vi "Login.vi"(0 "reference in":refnum<class "Login_Dialog.lvclass">, 11 "error in (no error)":errorcluster) -> (4 "reference in":refnum<class "Login_Dialog.lvclass">, 6 "User":string, 8 "Valid":bool, 10 "Rights":string[](array[string]), 13 "Password":string, 14 "Cancelled":bool, 15 "error out":errorcluster)   [LabVIEW 2022 SP3, in "Login_Dialog.lvlib" / "Login_Dialog.lvclass"]
uses:
  Login_Dialog.lvclass
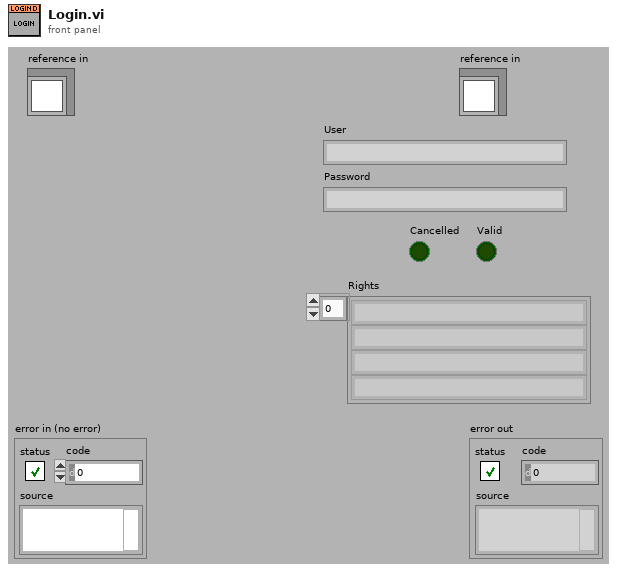
[diagram p1: front panel]
types:
  T1 = typedef "Login_Dialog.lvlib/Login_Dialog.lvclass/ObjectAttributes.ctl" = cluster{"Config":T2, "User":string, "LoggedIn":bool, "Users":string[][]}
  T2 = typedef "Login_Dialog.lvlib/Login_Dialog.lvclass/Config.ctl" = cluster{"default":string}
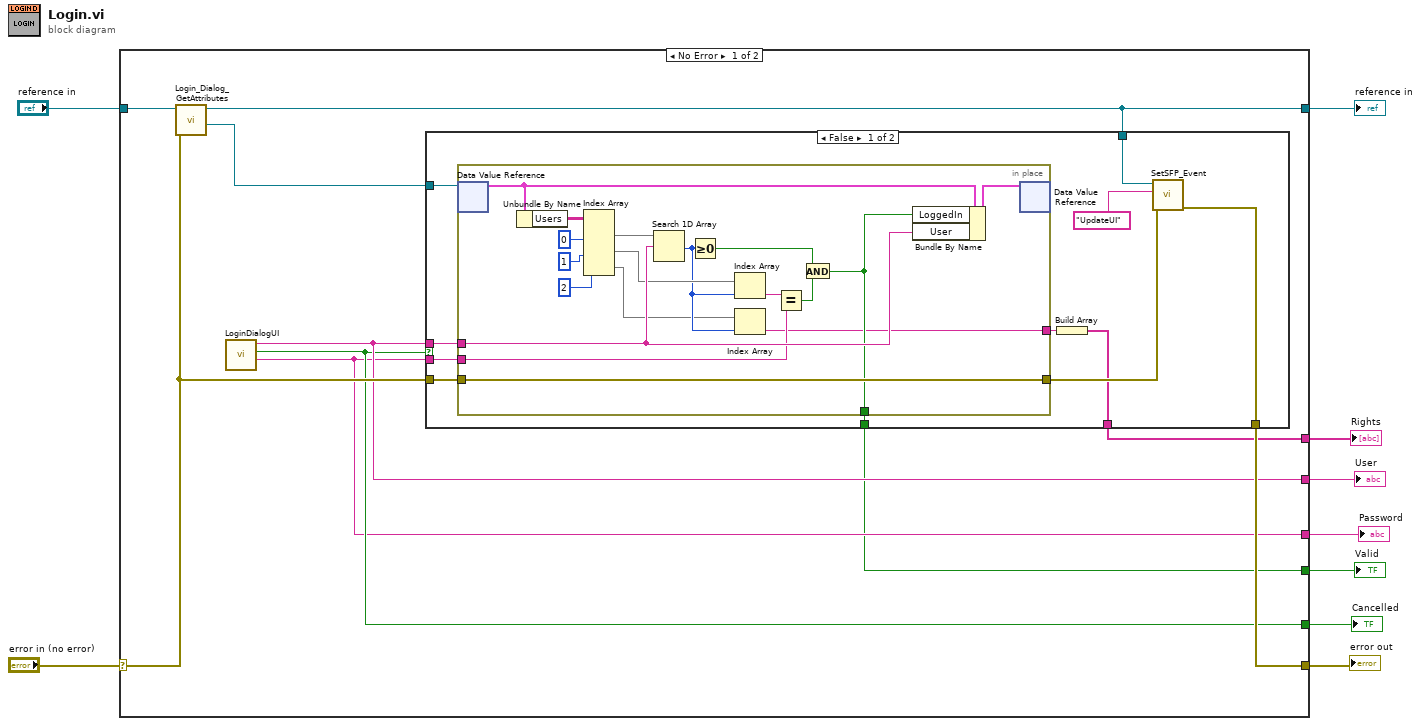
[diagram p0: block diagram]
diagram:
  n1 = case shown="No Error" "error in (no error)" {
    selector: "error in (no error)" -> [w15 w51]
    tunnel: [w16 w51] -> w8
    tunnel: [w17 w50] -> w6
    tunnel: "reference in" -> [w19 w50]
    tunnel: [w14 _] -> w5
    tunnel: [w13 _] -> w4
    tunnel: [w12 _] -> w3
    tunnel: [w11 _] -> w2
    tunnel: [w10 _] -> w1
    frame No Error {
      n2 = call "Login_Dialog_GetAttributes.vi"("error in (no error)"=w15, "reference in"=w19) -> ("DataRef"=w18:refnum<data-value>, "reference out"=w17:refnum<class "Login_Dialog.lvclass">)  [unwired: 6 in, 2 out]
      n3 = call "LoginDialogUI.vi"() -> ("PWord"=w12:string, "Cancelled"=w13:bool, "UserName"=w14:string)  [unwired: 9 in]
      n4 = case shown="False" w13 {
        tunnel: w18 -> [w30 _]
        tunnel: w14 -> [w29 _]
        tunnel: w17 -> [w28 _]
        tunnel: w15 -> [w26 w49]
        tunnel: [w24 w49] -> w16
        tunnel: w12 -> [w23 _]
        tunnel: [w22 _] -> w11
        tunnel: [w20 _] -> w10
        frame False {
          n5 = in-place {
            in-place-border: w29 -> [w42]
            in-place-border: [w47] -> w25
            in-place-border: w26 -> [w47]
            in-place-border: w23 -> [w38]
            in-place-border: [w35] -> w22
            in-place-border: [w31] -> w21
            n6 = in-place-dvr #1(w30) -> (w46:T1)  [unwired: 1 out]
            n7 = Unbundle By Name(w46) -> ("Users"=w45:string[][])
            n8 = Index Array(array=w45, index (col) #1=0 ("disabled index (col)"), index (col) #2=1 ("index (col)"), index (col) #3=2 ("index (col)")) -> (element #1=w43:string[], element #2=w40:string[], element #3=w32:string[])  [unwired: 3 in]
            n9 = Search 1D Array(1D array=w43, element=w42) -> (index of element=w33:i32)  [unwired: 1 in]
            n10 = Greater Or Equal To 0?(x=w33) -> (x >= 0?=w37:bool)
            n11 = Index Array(array=w40, index=w33) -> (element=w39:string)
            n12 = Index Array(array=w32, index=w33) -> (element=w31:string)
            n13 = Equal?(x=w39, y=w38) -> (x = y?=w36:bool)
            n14 = And(x=w37, y=w36) -> (x .and. y?=w35:bool)
            n15 = Bundle By Name(cluster=w46, "LoggedIn"=w35, "User"=w42) -> (w48:T1)
            n16 = in-place-dvr #1(w48) -> ()  [unwired: 2 out]
          }
          n17 = Build Array(w21) -> (w20:string[])
          n18 = call-dynamic "SetSFP_Event.vi"("error in (no error)"=w25, "msg"="UpdateUI", "reference in"=w28) -> ("error out"=w24:errorcluster)  [unwired: 7 in, 1 out]
        }
        frame True {
        }
      }
    }
    frame Error {
    }
  }
  "error out" <- w8
  "reference in" <- w6
  "User" <- w5
  "Rights" <- w1
  "Valid" <- w2
  "Cancelled" <- w4
  "Password" <- w3
